vi "Leading Frequency Estimator.vi"() -> ()   [LabVIEW 2023]
doc: "This example demonstrates how to extract the leading frequency components in exponentially-damped sinusoids by using the TSA Capon Frequency Estimator VI. You can compare the power magnitudes and frequencies that this examples returns. The power magnitudes and frequencies are computed by using the Capon method.\n\n<b>Instructions:</b>\n1) Run this VI.\n2) Specify the frequencies of the simulated sinusoids.\n3) Observe the detected frequencies and powers at these specified frequencies to determine the leading frequency."
uses:
  <vilib>/addons/Time Series Analysis/Modeling and Prediction.llb/TSA Capon Frequency Estimator (Waveform).vi
  <vilib>/measure/NI_MABase.lvlib
  <vilib>/addons/_Advanced Signal Processing/NI_AdvSigProcTSA.lvlib
panel:
  in  "Amplitude 2 (a2)":dbl=1.0 format="%.2p"
  in  "Amplitude 1 (a1)":dbl=2.0 format="%.2p"
  in  "FIR filter length":i32=64
  in  "Frequency band (Hz)":cluster{"Start":dbl, "End":dbl}={"Start"=0.0, "End"=250.0}
  in  "Gaussian noise":dbl=0.1 min=0.0 step=0.1
  in  "stop":bool
  out "a1*sin(2p*f1) + a2*sin(2p*f2) + Gaussian Noise":waveform(dbl)(graph)
  out "Frequencies (Hz)":dbl[](array[numeric])
  out "Power":dbl[](array[numeric])
  in  "f2 (Hz)":dbl=130.0 format="%.0p"
  in  "f1 (Hz)":dbl=120.0 format="%.0p"
  # "Overview: Demonstrates how to extract the leading frequency components in exponentially-damped sinusoids by using the TSA Capon Frequency Estimator VI.\nRequirements: LabVIEW Full Development System, Advanced Signal Processing Toolkit\nInstructions: \n1. Run this VI.\n2. Specify the frequencies of the simulated sinusoids.\n3. Observe the detected frequencies and powers at these specified frequencies to determine the leading frequency.\n4.  Click Stop to stop the VI."
  # "Signal Simulation"
  # "Settings"
  # "Estimated Parameters"
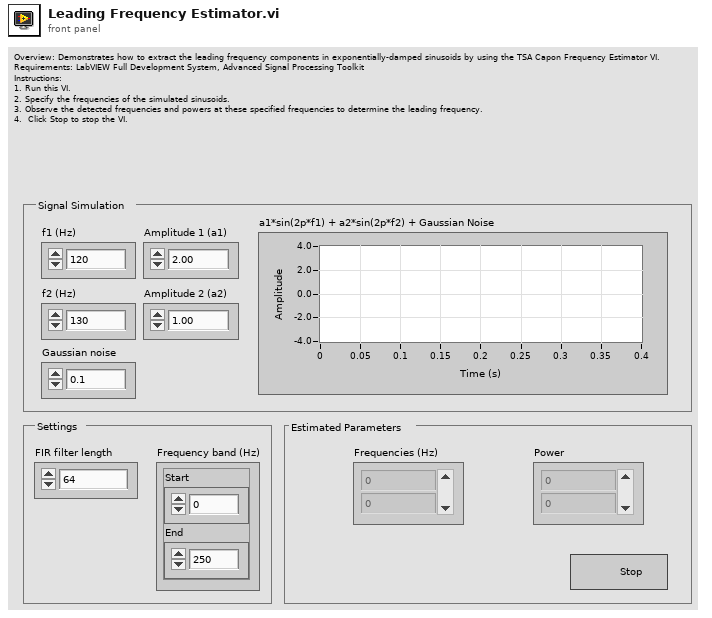
[diagram p1: front panel]
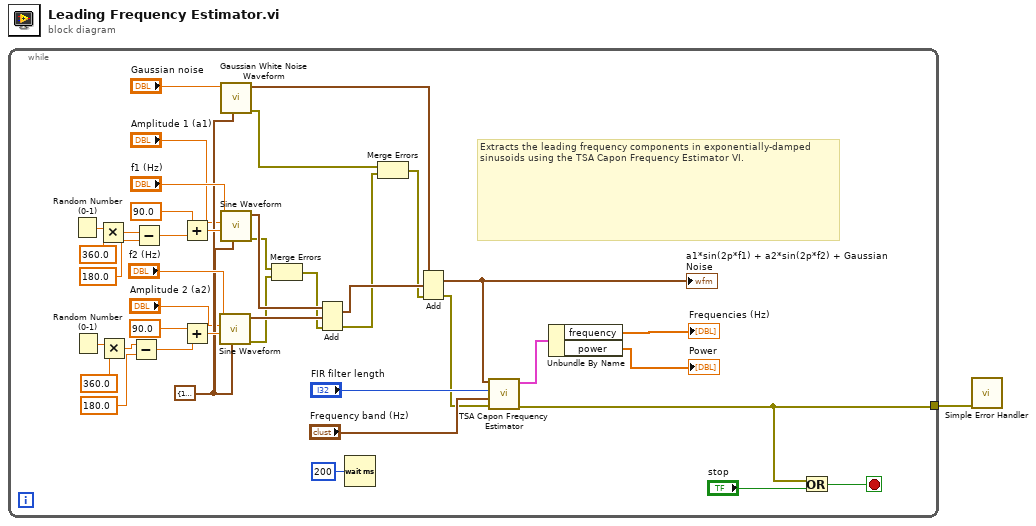
[diagram p0: block diagram]
diagram:
  n1 = while {
    tunnel: [w9] -> w1
    stop <- w24 stop-if-true
    w22 = cluster{"Fs":dbl, "#s":dbl} {"Fs"=1000.0, "#s"=400.0} ("Sampling Info")
    # "Extracts the leading frequency components in exponentially-damped sinusoids using the TSA Capon Frequency Estimator VI."
    n2 = Random Number (0-1)() -> (number: 0 to 1=w39:dbl)
    n3 = Random Number (0-1)() -> (number: 0 to 1=w37:dbl)
    n4 = Multiply(x=w39, y=360.0) -> (x*y=w34:dbl)
    n5 = Multiply(x=w37, y=360.0) -> (x*y=w32:dbl)
    n6 = Subtract(x=w32, y=180.0) -> (x-y=w30:dbl)
    n7 = Subtract(x=w34, y=180.0) -> (x-y=w35:dbl)
    n8 = Add(x=90.0, y=w35) -> (x+y=w42:dbl)
    n9 = Add(x=90.0, y=w30) -> (x+y=w41:dbl)
    n10 = call <vilib>:"Sine Waveform.vi"("sampling info"=w22, "phase"=w41, "amplitude"="Amplitude 2 (a2)", "frequency"="f2 (Hz)") -> ("error out"=w7:errorcluster, "signal out"=w11:waveform(dbl))  [unwired: 3 in, 3 out]
    n11 = call <vilib>:"Gaussian White Noise Waveform.vi"("sampling info"=w22, "standard deviation"="Gaussian noise") -> ("error out"=w5:errorcluster, "signal out"=w12:waveform(dbl))  [unwired: 3 in, 5 out]
    n12 = call <vilib>:"Sine Waveform.vi"("sampling info"=w22, "phase"=w42, "amplitude"="Amplitude 1 (a1)", "frequency"="f1 (Hz)") -> ("error out"=w8:errorcluster, "signal out"=w10:waveform(dbl))  [unwired: 3 in, 3 out]
    n13 = Merge Errors(w8, w7) -> (w6:errorcluster)
    n14 = Add(1:w11, 2:w10, 4:w6) -> (0:w26:waveform(dbl), 3:w4:errorcluster)
    n15 = Wait (ms)(milliseconds to wait=u32 200 ("millisecond multiple")) -> ()  [unwired: 1 out]
    n16 = Merge Errors(w5, w4) -> (w3:errorcluster)
    n17 = Add(1:w26, 2:w12, 4:w3) -> (0:w13:waveform(dbl), 3:w2:errorcluster)
    "a1*sin(2p*f1) + a2*sin(2p*f2) + Gaussian Noise" <- w13
    n18 = call-poly <vilib>:"TSA Capon Frequency Estimator.vi"("error in (no error)"=w2, "frequency band"="Frequency band (Hz)", "FIR filter length"="FIR filter length", "Xt"=w13) -> ("error out"=w9:errorcluster, "frequency components"=w18:cluster{"frequency":dbl[], "power":dbl[]})  [unwired: 1 in, 5 out]
    n19 = Unbundle By Name(w18) -> ("frequency"=→"Frequencies (Hz)":dbl[], "power"=→"Power":dbl[])
    n20 = Or(x=w9, y="stop") -> (x .or. y?=w24:bool)
  }
  n21 = call <vilib>:"Simple Error Handler.vi"("error in (no error)"=w1) -> ()  [unwired: 1 in, 8 out]
